vi "Unflatten.vi"(8 "error in (no error)":errorcluster, 9 "timeout in":bool, 10 "Data in":T1[](array[typedef]), 11 "CIFFifoCAN in":refnum<class "CIF_NIChn_Fifo_Power.lvclass">) -> (0 "error out":errorcluster, 2 "Data out":T1[](array[typedef]), 3 "CIFFifoCAN out":refnum<class "CIF_NIChn_Fifo_Power.lvclass">, 4 "Header":T2)   [LabVIEW 2021, in "CIF_NIChn_Fifo_Power.lvclass"]
uses:
  CIF_NIChn_Fifo_Power.lvclass
  CIF_NIChn_Fifo_Power.lvclass/CIF_NIChn_Fifo_Power.ctl
  ChannelCommon/CIFFIFO/CIFfifo.lvclass
  ChannelCommon/typedef/FIFO Header.ctl
  ChannelCommon/ChannelCommon.lvlib
  ChannelCommon/typedef/Datatype Waveform.ctl
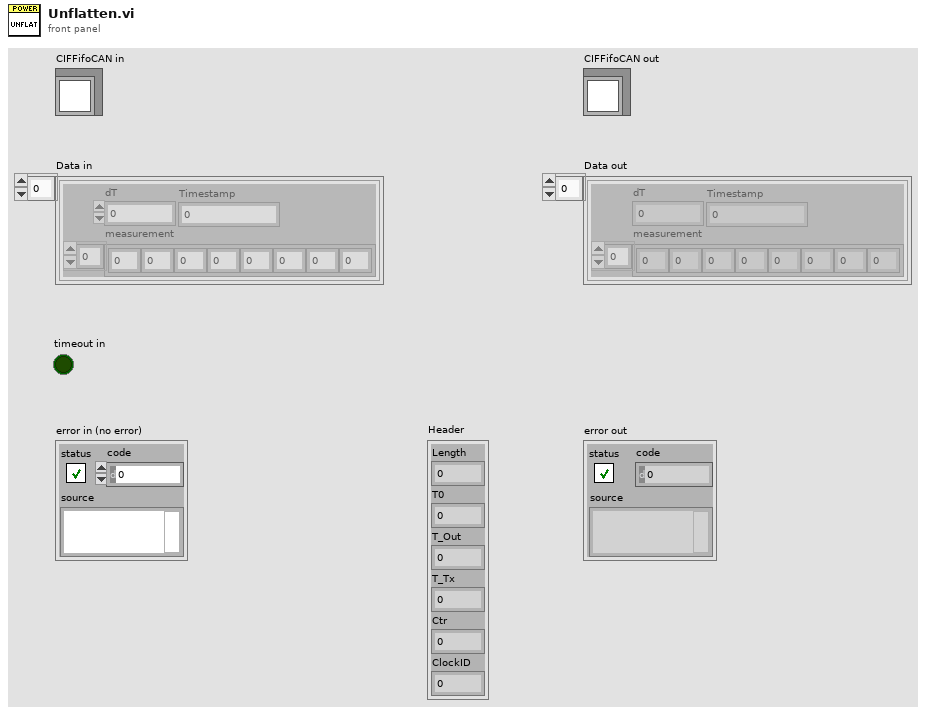
[diagram p1: front panel]
types:
  T1 = typedef "ChannelCommon.lvlib/Datatype Waveform.ctl" = cluster{"measurement":dbl[], "dT":dbl, "Timestamp":u64}
  T2 = typedef "ChannelCommon.lvlib/FIFO Header.ctl" = cluster{"Length":u64, "T0":u64, "T_Out":u64, "T_Tx":u64, "Ctr":u64, "ClockID":u8}
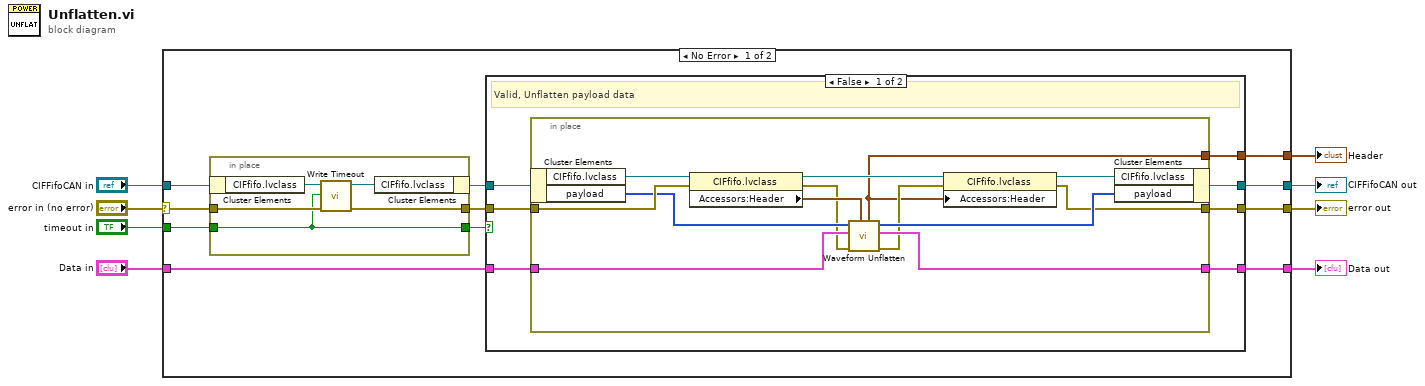
[diagram p0: block diagram]
diagram:
  n1 = case shown="No Error" "error in (no error)" {
    selector: "error in (no error)" -> [w18 w48]
    tunnel: [w11 w48] -> w7
    tunnel: [w12 w47] -> w5
    tunnel: "CIFFifoCAN in" -> [w19 w47]
    tunnel: "timeout in" -> [w17 _]
    tunnel: [w14 _] -> w2
    tunnel: [w13 _] -> w3
    tunnel: "Data in" -> [w9 _]
    frame No Error {
      n2 = in-place {
        in-place-border: w18 -> [w44]
        in-place-border: [w43] -> w16
        in-place-border: w17 -> [w42]
        in-place-border: [w42] -> w10
        n3 = in-place-cluster #1(w19) -> ("CIFfifo.lvclass"=w46:refnum<class "CIFfifo.lvclass">)
        n4 = call "Write Timeout.vi"("error in (no error)"=w44, "Timeout"=w42, "CIFFIFO in"=w46) -> ("error out"=w43:errorcluster, "CIFFIFO out"=w45:refnum<class "CIFfifo.lvclass">)  [unwired: 7 in]
        n5 = in-place-cluster #1("CIFfifo.lvclass"=w45) -> (w15:refnum<class "CIF_NIChn_Fifo_Power.lvclass">)
      }
      n6 = case shown="False" w10 {
        tunnel: w16 -> [w26 w40]
        tunnel: w15 -> [w25 w41]
        tunnel: [w24 _] -> w14
        tunnel: [w23 _] -> w13
        tunnel: [w22 w41] -> w12
        tunnel: [w21 w40] -> w11
        tunnel: w9 -> [w20 _]
        frame False {
          # "Valid, Unflatten payload data"
          n7 = in-place {
            in-place-border: w26 -> [w39]
            in-place-border: [w33] -> w24
            in-place-border: [w27] -> w23
            in-place-border: [w28] -> w21
            in-place-border: w20 -> [w34]
            n8 = in-place-cluster #2(w25) -> ("CIFfifo.lvclass"=w37:refnum<class "CIFfifo.lvclass">, "payload"=w32:u8[])
            n9 = property class="CIFfifo.lvclass"(reference=w37, error in=w39) -> (reference out=w38:refnum<class "CIFfifo.lvclass">, error out=w30:errorcluster, "Accessors:Header"=w31:T2)
            n10 = call "Waveform Unflatten.vi"("Header in"=w31, "error in (no error)"=w30, "Data in in"=w34, "Flatten Data in"=w32) -> ("error out"=w29:errorcluster, "Data out"=w33:T1[], "Flatten Data out"=w35:u8[], "Header out"=w27:T2)  [unwired: 4 in]
            n11 = property class="CIFfifo.lvclass"(reference=w38, error in=w29, "Accessors:Header"=w27) -> (reference out=w36:refnum<class "CIFfifo.lvclass">, error out=w28:errorcluster)
            n12 = in-place-cluster #2("CIFfifo.lvclass"=w36, "payload"=w35) -> (w22:refnum<class "CIF_NIChn_Fifo_Power.lvclass">)
          }
        }
        frame True {
          # "Timeout"
        }
      }
    }
    frame Error {
    }
  }
  "error out" <- w7
  "CIFFifoCAN out" <- w5
  "Header" <- w3
  "Data out" <- w2
